vi "niDAQmx Attach gRPC Task.vi"(0 "task name":string, 11 "error in":errorcluster) -> (4 "task out":refnum<class "Session Factory.lvclass">, 15 "error out":errorcluster)   [LabVIEW 2021, in "Session Management niDAQmx.lvlib" / "Session Factory.lvclass"]
doc: "Attaches to an existing niDAQmx task on the specified NI gRPC Device Server. Returns a session factory object to be used in all subsequent niDAQmx client wrapper VI calls."
uses:
  Session Factory.lvclass
  NI_DAQmx_client/RPC Messages/nidaqmx_grpc_CreateTaskRequest.ctl
  NI_DAQmx_client/RPC Messages/nidevice_grpc_SessionInitializationBehavior.ctl
  <vilib>/gRPC/Generated APIs/ni/measurementlink/discovery/v1/RPC Messages/ni_measurementlink_discovery_v1_ResolveServiceRequest.ctl
  Session Factory.lvclass/Session Factory.ctl
  NI_DAQmx_client/NI_DAQmx_client.lvlib
  <vilib>/gRPC/Generated APIs/ni/measurementlink/discovery/v1/ni.measurementlink.discovery.v1.api.lvlib
  <vilib>/Plug-In SDKs/Clients/Discovery V1/NI Discovery V1 Client.lvlib
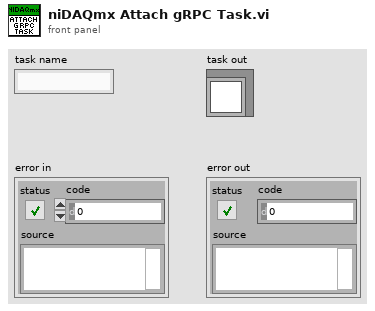
[diagram p1: front panel]
types:
  T1 = typedef "NI_DAQmx_client.lvlib/nidevice_grpc_SessionInitializationBehavior.ctl" = enum32{"SESSION_INITIALIZATION_BEHAVIOR_UNSPECIFIED", "SESSION_INITIALIZATION_BEHAVIOR_INITIALIZE_NEW", "SESSION_INITIALIZATION_BEHAVIOR_ATTACH_TO_EXISTING"}
  T2 = typedef "ni.measurementlink.discovery.v1.api.lvlib/ni_measurementlink_discovery_v1_ResolveServiceRequest.ctl" = cluster{"provided_interface":string, "service_class":string, "deployment_target":string, "version":string}
  T3 = typedef "NI_DAQmx_client.lvlib/nidaqmx_grpc_CreateTaskRequest.ctl" = cluster{"session_name":string, "initialization_behavior":T1}
  T4 = typedef "ni.measurementlink.discovery.v1.api.lvlib/ni_measurementlink_discovery_v1_ServiceLocation.ctl" = cluster{"location":string, "insecure_port":string, "ssl_authenticated_port":string}
  T5 = typedef "grpc-lvsupport-release.lvlib/grpcId.ctl" = u64
  T6 = typedef "NI_DAQmx_client.lvlib/nidaqmx_grpc_CreateTaskResponse.ctl" = cluster{"status":i32, "task":T7, "new_session_initialized":bool}
  T7 = typedef "NI_DAQmx_client.lvlib/nidevice_grpc_Session.ctl" = cluster{"nidevice_grpc_Session_session":refnum<class "nidevice_grpc_Session_session.lvclass">}
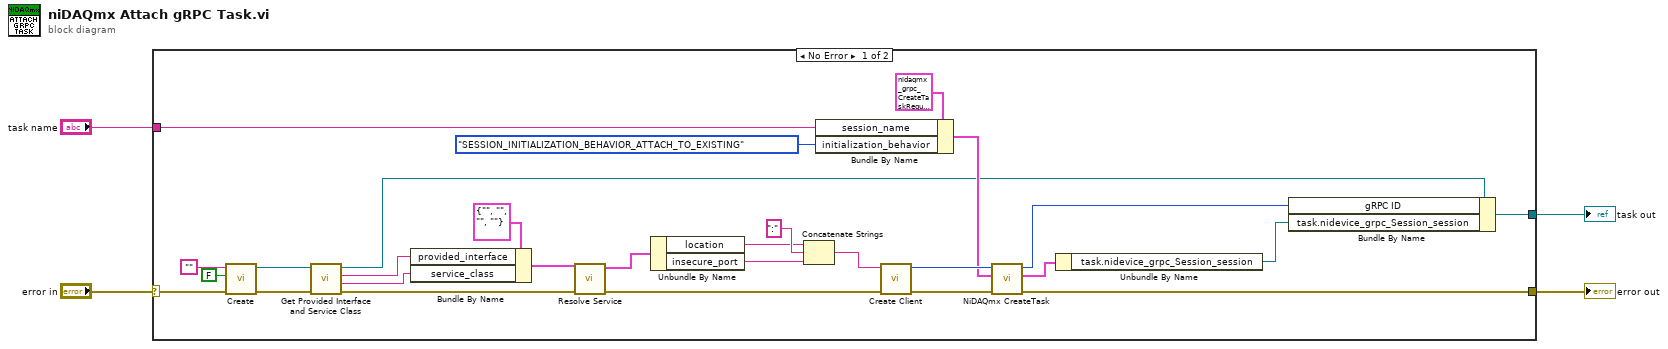
[diagram p0: block diagram]
diagram:
  n1 = case shown="No Error" "error in" {
    selector: "error in" -> [w18 w33]
    tunnel: [w30 w33] -> w3
    tunnel: "task name" -> [w23 _]
    tunnel: [w6 _] -> w1
    frame No Error {
      n2 = call "Create.vi"("error in"=w18, "reset"=FALSE, "option string"="") -> ("error out"=w15:errorcluster, "session factory out"=w13:refnum<class "Session Factory.lvclass">)  [unwired: 7 in]
      n3 = call-dynamic "Get Provided Interface and Service Class.vi"("error in"=w15, "session factory in"=w13) -> ("error out"=w14:errorcluster, "service class"=w11:string, "provided interface"=w12:string, "session factory out"=w10:refnum<class "Session Factory.lvclass">)  [unwired: 6 in]
      n4 = Bundle By Name(cluster=T2 {"provided_interface"="", "service_class"="", "deployment_target"="", "version"=""} ("request data"), "provided_interface"=w12, "service_class"=w11) -> (w20:T2)
      n5 = call <vilib>:"Resolve Service.vi"("error in"=w14, "request data"=w20) -> ("error out"=w21:errorcluster, "response data"=w19:T4)  [unwired: 8 in]
      n6 = Unbundle By Name(w19) -> ("location"=w28:string, "insecure_port"=w27:string)
      n7 = Concatenate Strings(w28, ":" ("string"), w27) -> (w26:string)
      n8 = Bundle By Name(cluster=T3 {"session_name"="", "initialization_behavior"=enum."SESSION_INITIALIZATION_BEHAVIOR_INITIALIZE_NEW"} ("Request Data"), "session_name"=w23, "initialization_behavior"=nidevice_grpc_SessionInitializationBehavior."SESSION_INITIALIZATION_BEHAVIOR_ATTACH_TO_EXISTING") -> (w24:T3)
      n9 = call "Create Client.vi"("error in"=w21, "address"=w26) -> ("error out"=w32:errorcluster, "gRPC ID Out"=w31:T5)  [unwired: 8 in]
      n10 = call "NiDAQmx CreateTask.vi"("error in"=w32, "Request Data"=w24, "gRPC ID"=w31) -> ("error out"=w30:errorcluster, "Response Data"=w8:T6, "gRPC ID out"=w9:T5)  [unwired: 6 in]
      n11 = Unbundle By Name(w8) -> ("task.nidevice_grpc_Session_session"=w7:refnum<class "nidevice_grpc_Session_session.lvclass">)
      n12 = Bundle By Name(cluster=w10, "gRPC ID"=w9, "task.nidevice_grpc_Session_session"=w7) -> (w6:refnum<class "Session Factory.lvclass">)
    }
    frame Error {
    }
  }
  "error out" <- w3
  "task out" <- w1
